vi "Set Cell (String).vi"(6 "Column":i32, 7 "Value":string, 8 "error in (no error)":errorcluster, 9 "Row":i32, 10 "Sheet Reference":refnum<k24>) -> (0 "error out":errorcluster, 2 "Sheet Reference out":refnum<k24>)   [LabVIEW 2013]
uses:
  C:/PhaeronGit/LVNPOI/Resources/NPOI 2.1.1 dotnet2/NPOI.dll
  Resources/NPOI 2.1.1 dotnet2/NPOI.dll
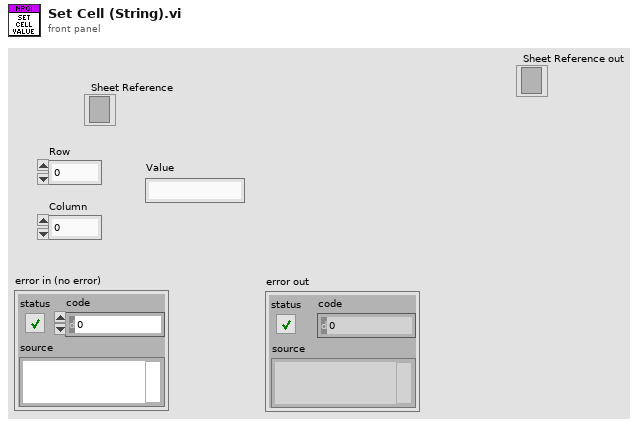
[diagram p1: front panel]
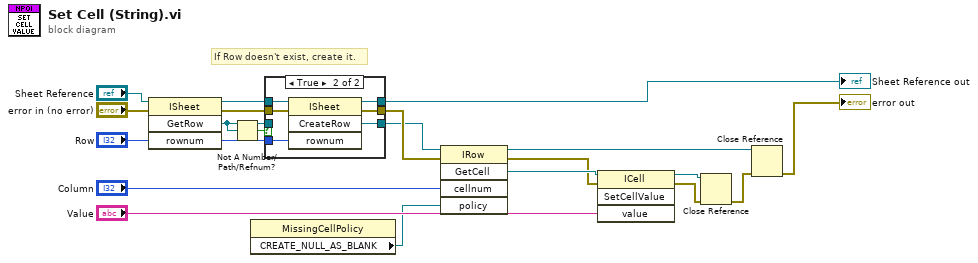
[diagram p0: block diagram]
diagram:
  # "If Row doesn't exist, create it."
  n1 = invoke class="ISheet" method="GetRow"(reference="Sheet Reference", error in="error in (no error)", "rownum"="Row") -> (reference out=w8:refnum<k24>, error out=w9:errorcluster, "GetRow"=w11:refnum<k24>)  [unwired: 1 in, 1 out]
  n2 = Not A Number/Path/Refnum?(number/path/refnum=w11) -> (NaN/Path/Refnum?=w10:bool)
  n3 = property class="MissingCellPolicy"() -> ("CREATE_NULL_AS_BLANK"=w1:refnum<k24>)  [unwired: 2 in, 2 out]
  n4 = case shown="True" w10 {
    tunnel: w8 -> [w23 w29]
    tunnel: w9 -> [w22 w28]
    tunnel: [w22 w27] -> w3
    tunnel: [w23 w26] -> w4
    tunnel: "Row" -> [_ w25]
    tunnel: [w21 w24] -> w2
    tunnel: w11 -> [w21 _]
    frame False {
    }
    frame True {
      n5 = invoke class="ISheet" method="CreateRow"(reference=w29, error in=w28, "rownum"=w25) -> (reference out=w26:refnum<k24>, error out=w27:errorcluster, "CreateRow"=w24:refnum<k24>)  [unwired: 1 in, 1 out]
    }
  }
  "Sheet Reference out" <- w4
  n6 = invoke class="IRow" method="GetCell"(reference=w2, error in=w3, "cellnum"="Column", "policy"=w1) -> (reference out=w20:refnum<k24>, error out=w17:errorcluster, "GetCell"=w18:refnum<k24>)  [unwired: 1 in, 2 out]
  n7 = invoke class="ICell" method="SetCellValue"(reference=w18, error in=w17, "value"="Value") -> (reference out=w16:refnum<k24>, error out=w15:errorcluster)  [unwired: 1 in, 2 out]
  n8 = Close Reference(reference=w16, error in (no error)=w15) -> (error out=w14:errorcluster)
  n9 = Close Reference(reference=w20, error in (no error)=w14) -> (error out=→"error out":errorcluster)
